vi "DetParsEng.vi"() -> ()   [LabVIEW 2014]
uses:
  DetectorGlobals.vi
panel:
  in  "OK":bool caption="Boolean"
  in  "Apply":bool caption="Boolean"
  in  "Quit":bool
  in  "Tab Control":T1(tab)
  in  "Underscan\nRows":i32 min=0 step=1
  in  "Underscan\nCols":i32 min=0 step=1
  in  "Last \nColumn":i32=4096 min=1 step=1
  in  "Last\nRow":i32=4096 min=1 step=1
  in  "Row\nBin":i32=3 min=1 max=100 step=1
  in  "Column\nBin":i32=5 min=1 max=100 step=1
  in  "Overscan\nRows":i32 min=0
  in  "Overscan\nCols":i32=20 min=0
  in  "First \nColumn":i32=1 min=1 step=1
  in  "First\nRow":i32=1 min=1 step=1
  in  "NPframetransfer":i32 min=0
  in  "darkCols":i32=5 min=0 step=1
  in  "darkRows":i32 min=0 step=1
  in  "DeviceCols":i32=4096
  in  "DeviceRows":i32=4096
  in  "NumAmpsY":u8=2 min=1
  in  "NumAmpsX":u8=2 min=1
  in  "AmpConfig":string="01010101" caption="Amplifier Configuration String"
  in  "NumDetY":u8=2 min=1
  in  "NumDetX":u8=2 min=1
  in  "Video Gain":i32 min=0 step=1
  in  "Close":bool caption="Boolean"
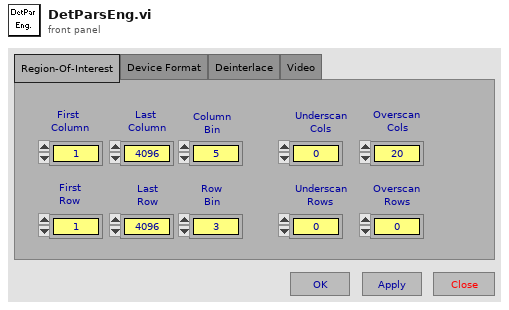
[diagram p1: front panel]
types:
  T1 = enum32{"Region-Of-Interest", "Device Format", "Deinterlace", "Video"}
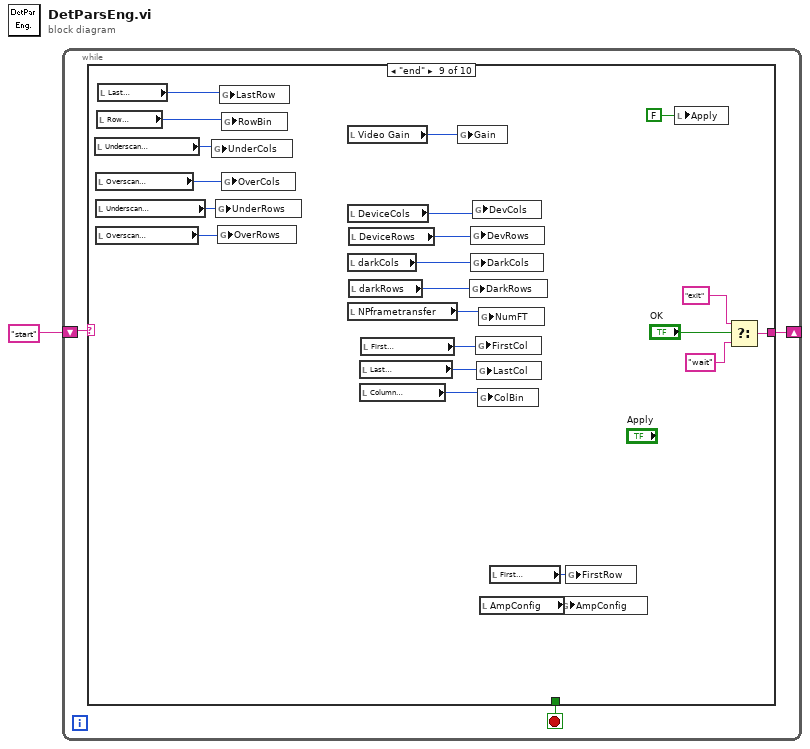
[diagram p0: block diagram]
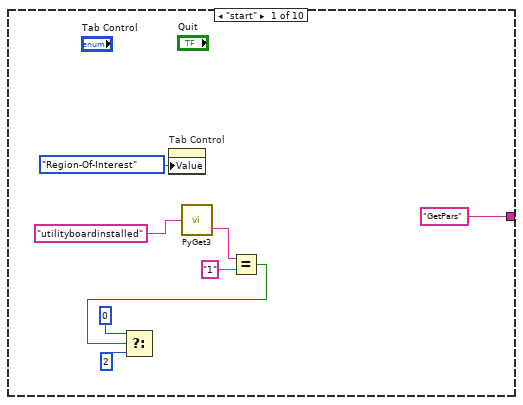
[diagram p2: hidden frame]
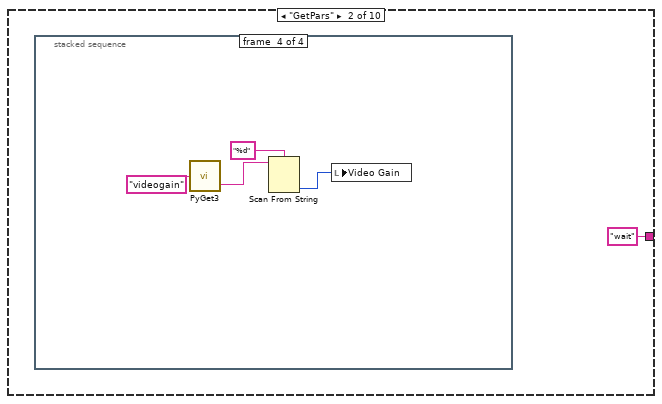
[diagram p3: hidden frame]
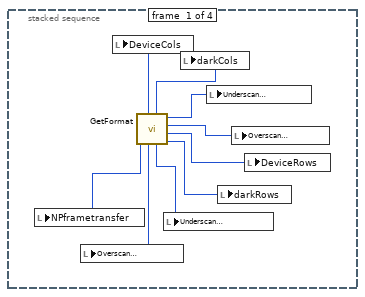
[diagram p4: hidden frame]
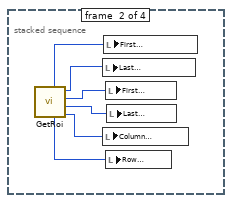
[diagram p5: hidden frame]
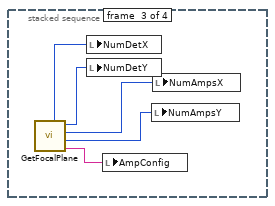
[diagram p6: hidden frame]
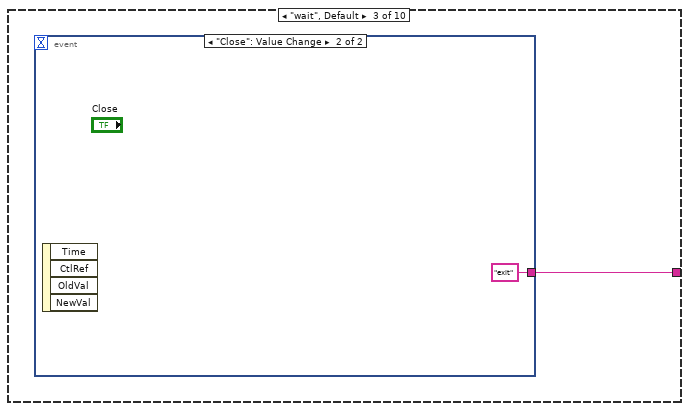
[diagram p7: hidden frame]
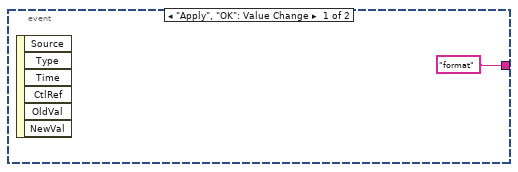
[diagram p8: hidden frame]
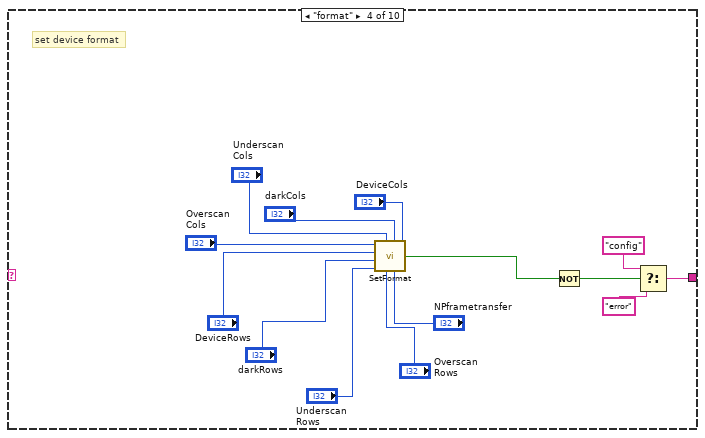
[diagram p9: hidden frame]
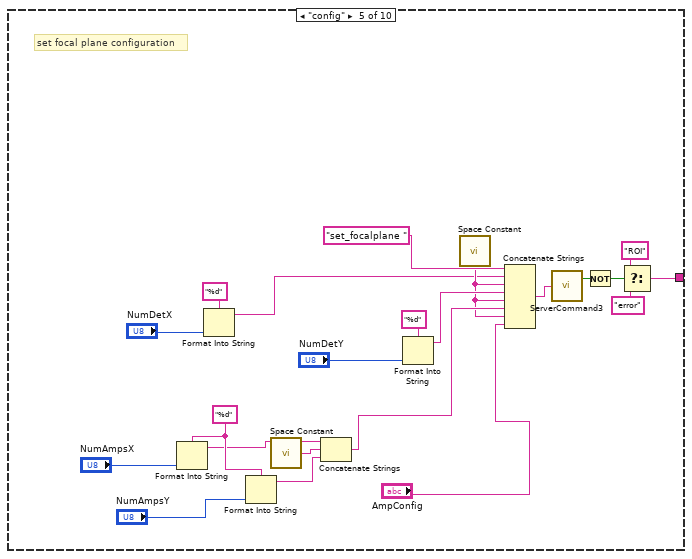
[diagram p10: hidden frame]
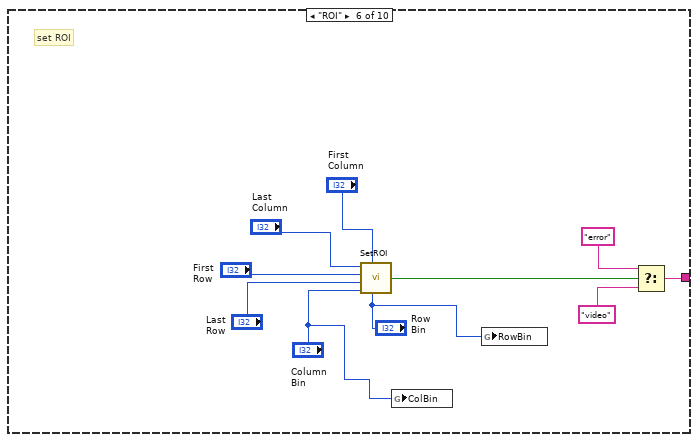
[diagram p11: hidden frame]
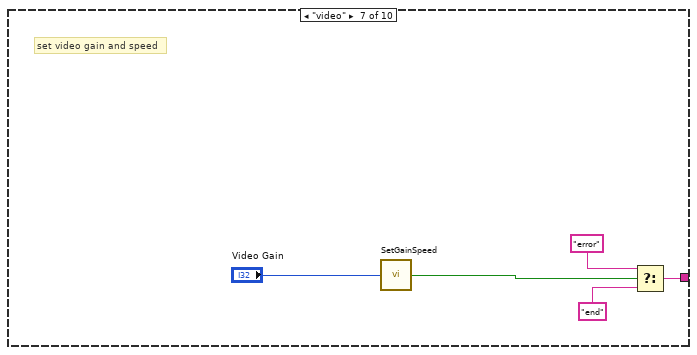
[diagram p12: hidden frame]
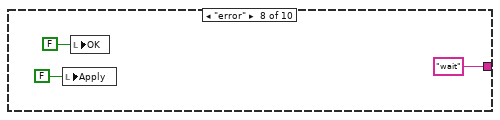
[diagram p13: hidden frame]
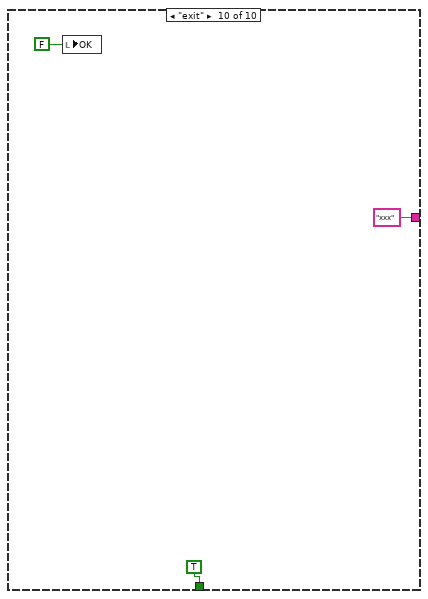
[diagram p14: hidden frame]
diagram:
  n1 = while {
    shift-right: [w3] -> _
    shift-left: "start" -> [w4]
    stop <- w2 stop-if-true
    n2 = case shown="\"end\"" w4 {
      tunnel: ["GetPars" "wait" w38 w47 w74 w82 w89 "wait" w116 "xxx"] -> w3
      tunnel: [_ _ _ _ _ _ _ _ _ TRUE] -> w2
      frame "start" {
        n3 = property on="Tab Control" class="TabCtl (strict)"("Value"=T1."Region-Of-Interest" ("Tab Control")) -> ()  [unwired: 2 in, 2 out]
        n4 = call "PyGet3.vi"("Attribute"="utilityboardinstalled") -> ("Reply"=w7:string)  [unwired: 1 out]
        n5 = Equal?(x=w7, y="1") -> (x = y?=w5:bool)
        n6 = Select(t=0, s=w5, f=2) -> ()  [unwired: 1 out]
      }
      frame "GetPars" {
        n7 = stacked-sequence {
          frame #0 {
            n8 = call "GetFormat.vi"() -> ("NPdark"=w17:i32, "NPtotal"=w18:i32, "NSoverscan"=w19:i32, "NSunderscan"=w20:i32, "NPunderscan"=w15:i32, "NSdark"=w21:i32, "NPoverscan"=w14:i32, "NStotal"=w22:i32, "NPframetransfer"=w16:i32)  [unwired: 3 in]
            n9 = local write "NPframetransfer"(w16) -> ()
            n10 = local write "Overscan\nRows"(w14) -> ()
            n11 = local write "DeviceCols"(w22) -> ()
            n12 = local write "Underscan\nRows"(w15) -> ()
            n13 = local write "darkCols"(w21) -> ()
            n14 = local write "Underscan\nCols"(w20) -> ()
            n15 = local write "darkRows"(w17) -> ()
            n16 = local write "Overscan\nCols"(w19) -> ()
            n17 = local write "DeviceRows"(w18) -> ()
          }
          frame #1 {
            n18 = call "GetRoi.vi"() -> ("FirstCol"=w23:i32, "RowBin"=w28:i32, "LastCol"=w24:i32, "FirstRow"=w25:i32, "LastRow"=w26:i32, "ColBin"=w27:i32)  [unwired: 1 in]
            n19 = local write "Last \nColumn"(w24) -> ()
            n20 = local write "Column\nBin"(w27) -> ()
            n21 = local write "First \nColumn"(w23) -> ()
            n22 = local write "First\nRow"(w25) -> ()
            n23 = local write "Row\nBin"(w28) -> ()
            n24 = local write "Last\nRow"(w26) -> ()
          }
          frame #2 {
            n25 = call "GetFocalPlane.vi"() -> ("NumDetX"=w32:i32, "NumDetY"=w31:i32, "NumAmpsX"=w30:i32, "NumAmpsY"=w29:i32, "AmpConfig"=w33:string)  [unwired: 2 in]
            n26 = local write "NumDetX"(w32) -> ()
            n27 = local write "NumDetY"(w31) -> ()
            n28 = local write "AmpConfig"(w33) -> ()
            n29 = local write "NumAmpsY"(w29) -> ()
            n30 = local write "NumAmpsX"(w30) -> ()
          }
          frame #3 {
            n31 = call "PyGet3.vi"("Attribute"="videogain") -> ("Reply"=w36:string)  [unwired: 1 out]
            n32 = Scan From String(format string="%d", input string=w36) -> (output 1=w34:i32)  [unwired: 3 in, 3 out]
            n33 = local write "Video Gain"(w34) -> ()
          }
        }
      }
      frame "wait", Default {
        n34 = event shown="[1] \"Close\": Value Change" {
          selector: _ -> [_ _]
          dyn-events: _ -> [_ _]
          timeout: _ -> [_ _]
          tunnel: ["format" "exit"] -> w38
          event "Apply", "OK": Value Change {
            n35 = event-data() -> ()  [unwired: 1 in, 6 out]
          }
          event "Close": Value Change {
            n36 = event-data() -> ()  [unwired: 1 in, 4 out]
          }
        }
      }
      frame "format" {
        # "set device format"
        n37 = call "SetFormat.vi"("NPframetransfer"="NPframetransfer", "NStotal"="DeviceCols", "NSdark"="darkCols", "NPoverscan"="Overscan\nRows", "NPunderscan"="Underscan\nRows", "NPdark"="darkRows", "NSunderscan"="Underscan\nCols", "NPtotal"="DeviceRows", "NSoverscan"="Overscan\nCols") -> ("Error"=w42:bool)  [unwired: 1 in]
        n38 = Not(x=w42) -> (.not. x?=w41:bool)
        n39 = Select(t="config", s=w41, f="error") -> (s? t:f=w47:string)
      }
      frame "config" {
        w73 = "%d" ("format string")
        # "set focal plane configuration"
        n40 = Format Into String(format string=w73, "NumAmpsX") -> (resulting string=w72:string)  [unwired: 2 in, 1 out]
        n41 = Format Into String(format string="%d", "NumDetX") -> (resulting string=w60:string)  [unwired: 2 in, 1 out]
        n42 = Format Into String(format string=w73, "NumAmpsY") -> (resulting string=w70:string)  [unwired: 2 in, 1 out]
        n43 = call <vilib>:"Space Constant.vi"() -> ("String"=w71:string)
        n44 = Concatenate Strings(w72, w71, w70) -> (w64:string)
        n45 = Format Into String(format string="%d", "NumDetY") -> (resulting string=w65:string)  [unwired: 2 in, 1 out]
        n46 = call <vilib>:"Space Constant.vi"() -> ("String"=w62:string)
        n47 = Concatenate Strings("set_focalplane " ("Command"), w60, w62, w65, w62, w64, w62, "AmpConfig") -> (w63:string)
        n48 = call "ServerCommand3.vi"("Command"=w63) -> ("Error"=w68:bool)  [unwired: 1 out]
        n49 = Not(x=w68) -> (.not. x?=w67:bool)
        n50 = Select(t="ROI", s=w67, f="error") -> (s? t:f=w74:string)
      }
      frame "ROI" {
        # "set ROI"
        n51 = call "SetROI.vi"("RowBIn"="Row\nBin", "FirstCol"="First \nColumn", "ColBin"="Column\nBin", "LastRow"="Last\nRow", "FirstRow"="First\nRow", "LastCol"="Last \nColumn") -> ("Error"=w79:bool)
        n52 = global write "DetectorGlobals.vi" "ColBin"("Column\nBin") -> ()
        n53 = global write "DetectorGlobals.vi" "RowBin"("Row\nBin") -> ()
        n54 = Select(t="error", s=w79, f="video") -> (s? t:f=w82:string)
      }
      frame "video" {
        # "set video gain and speed"
        n55 = call "SetGainSpeed.vi"("Gain"="Video Gain") -> ("Error"=w87:bool)
        n56 = Select(t="error", s=w87, f="end") -> (s? t:f=w89:string)
      }
      frame "error" {
        n57 = local write "Apply"(FALSE ("Apply")) -> ()
        n58 = local write "OK"(FALSE ("OK")) -> ()
      }
      frame "end" {
        n59 = local read "Underscan\nCols"() -> (w107:i32)
        n60 = local read "Overscan\nCols"() -> (w106:i32)
        n61 = local read "Underscan\nRows"() -> (w105:i32)
        n62 = local read "Overscan\nRows"() -> (w104:i32)
        n63 = local read "Row\nBin"() -> (w108:i32)
        n64 = local read "Last\nRow"() -> (w109:i32)
        n65 = global write "DetectorGlobals.vi" "UnderCols"(w107) -> ()
        n66 = global write "DetectorGlobals.vi" "UnderRows"(w105) -> ()
        n67 = global write "DetectorGlobals.vi" "OverRows"(w104) -> ()
        n68 = global write "DetectorGlobals.vi" "LastRow"(w109) -> ()
        n69 = global write "DetectorGlobals.vi" "RowBin"(w108) -> ()
        n70 = global write "DetectorGlobals.vi" "OverCols"(w106) -> ()
        n71 = local read "Video Gain"() -> (w112:i32)
        n72 = local read "DeviceCols"() -> (w103:i32)
        n73 = local read "darkCols"() -> (w101:i32)
        n74 = local read "NPframetransfer"() -> (w99:i32)
        n75 = local read "DeviceRows"() -> (w102:i32)
        n76 = local read "darkRows"() -> (w100:i32)
        n77 = local read "Last \nColumn"() -> (w97:i32)
        n78 = local read "Column\nBin"() -> (w98:i32)
        n79 = local read "First \nColumn"() -> (w96:i32)
        n80 = global write "DetectorGlobals.vi" "Gain"(w112) -> ()
        n81 = global write "DetectorGlobals.vi" "DarkRows"(w100) -> ()
        n82 = global write "DetectorGlobals.vi" "DevRows"(w102) -> ()
        n83 = global write "DetectorGlobals.vi" "DarkCols"(w101) -> ()
        n84 = global write "DetectorGlobals.vi" "DevCols"(w103) -> ()
        n85 = global write "DetectorGlobals.vi" "FirstCol"(w96) -> ()
        n86 = global write "DetectorGlobals.vi" "LastCol"(w97) -> ()
        n87 = global write "DetectorGlobals.vi" "ColBin"(w98) -> ()
        n88 = global write "DetectorGlobals.vi" "NumFT"(w99) -> ()
        n89 = local read "AmpConfig"() -> (w110:string)
        n90 = local read "First\nRow"() -> (w111:i32)
        n91 = global write "DetectorGlobals.vi" "AmpConfig"(w110) -> ()
        n92 = global write "DetectorGlobals.vi" "FirstRow"(w111) -> ()
        n93 = local write "Apply"(FALSE ("Apply")) -> ()
        n94 = Select(t="exit", s="OK", f="wait") -> (s? t:f=w116:string)
      }
      frame "exit" {
        n95 = local write "OK"(FALSE ("OK")) -> ()
      }
    }
  }
